vi "MainSimple.vi"() -> ()   [LabVIEW 2020]
uses:
  <vilib>/Platform/TimedLoop/XDataNode/timing_clust.ctl
  <vilib>/Platform/TimedLoop/XDataNode/nitl_modes.ctl
  <vilib>/Platform/TimedLoop/XDataNode/wakeup.ctl
  <vilib>/Platform/TimedLoop/XDataNode/loadnilvce.vi
  <vilib>/imath/engines/lvmath2/RunTimeEngine/Managers/WorkSpace/UID Generator.vi
  <vilib>/imath/engines/lvmath2/RunTimeEngine/RunTimeType/NIMS_RunTimeType_From StrictType (excl LVString).vi
  <instcachedir>/0/NIMS_RunTimeType_From StrictType (excl LVString)_283B1B2000484AAA8744D21CE97EA49F.lvgen/NIMS_RunTimeType_From StrictType (excl LVString)_283B1B2000484AAA8744D21CE97EA49F_000.vi
  <vilib>/imath/engines/lvmath2/RunTimeEngine/LocalVariableDefStatement/MC_LocalVariableDefStatement_Display.vi
  <vilib>/imath/engines/lvmath2/RunTimeEngine/BuiltInFunctions/round/NIMS_round(DBL-S).vi
  <vilib>/imath/engines/lvmath2/RunTimeEngine/RunTimeType/NIMS_RunTimeType_Set Source Original Bool.vi
  <vilib>/imath/engines/lvmath2/RunTimeEngine/Managers/SymbolTable/Clear UID.vi
  <vilib>/imath/engines/lvmath2/RunTimeEngine/NodeEndStatement/NIMS_NodeEndStatement_Output.vi
  <instcachedir>/0/NIMS_NodeEndStatement_Output_53EC0D466D134D7ABD903AC30B43404B.lvgen/NIMS_NodeEndStatement_Output_53EC0D466D134D7ABD903AC30B43404B_001.vi
  <instcachedir>/0/NIMS_NodeEndStatement_Output_53EC0D466D134D7ABD903AC30B43404B.lvgen/NIMS_NodeEndStatement_Output_53EC0D466D134D7ABD903AC30B43404B_010.vi
  <vilib>/imath/engines/lvmath2/RunTimeEngine/ErrorHandling/NIMS_Finalize Error.vi
  Global 2.vi
  <vilib>/platform/TimedLoop/XDataNode/XDataNode.xnode
  <vilib>/Platform/TimedLoop/XDataNode/XDNodeRunTimeDep.lvlib
  <vilib>/imath/engines/lvmath2/RunTimeEngine/Managers/SymbolTable/NIMS_WorkSpace.lvlib
panel:
  in  "AlphaX [rad]":dbl
  in  "AlphaY [rad]":dbl=1.57
  in  "SwimmerX [m]":dbl
  in  "SwimmerY [m]":dbl
  in  "SwimmerZ [m]":dbl
  in  "BMagnitude [T]":dbl=0.02
  out "LoopDuration [ms]":dbl=1.0
  out "Numeric":dbl=8325.0
  in  "Power On/Off":bool
  out "Power":bool
  out "VoltageSaturating":bool=TRUE
  out "Waveform Chart":dbl(graph)=-0.2668501091435667
  in  "ForwardRotationsPerSecond [Hz]":dbl=15.0
  in  "BackwardRotationsPerSecond [Hz]":dbl=-15.0
  in  "RotationsPerSecond [Hz]":dbl=-20.0
  in  "Bidirection":bool=TRUE
  out "RotationPerSecond[Hz]":dbl=94.24777499999999
  in  "Z_offset (m)":dbl
  in  "Search Rect (entire image)":T1={"Left"=256, "Top"=459, "Right"=496, "Bottom"=249, "Rotation"=0.0} {"Rotation" format="%.2f"; "Left" scale=0.0..1024.0; "Right" scale=0.0..1024.0}
  in  "Settings 4":T2={"Objects"=1, "Threshold"=95, "Reject Border"=FALSE, "Fill Holes"=FALSE, "Min Object Size"=TRUE, "Min Size"=25, "Max Object Size"=TRUE, "Max Size"=25000, "Show Search Area"=TRUE, "Show Center"=TRUE, "Show Bounding Box"=TRUE} {"Objects" items=["Bright Objects", "Dark Objects"]; "Threshold" min=1 max=999999999 step=1; "Max Size" min=1 max=999999999 step=1; "Min Size" min=1 max=999999999 step=1}
  out "Image 4":T3(plugin-control)
  in  "Settings 3":T2={"Objects"=1, "Threshold"=100, "Reject Border"=FALSE, "Fill Holes"=FALSE, "Min Object Size"=TRUE, "Min Size"=25, "Max Object Size"=TRUE, "Max Size"=25000, "Show Search Area"=FALSE, "Show Center"=TRUE, "Show Bounding Box"=TRUE} {"Objects" items=["Bright Objects", "Dark Objects"]; "Threshold" min=1 max=999999999 step=1; "Max Size" min=1 max=999999999 step=1; "Min Size" min=1 max=999999999 step=1}
  out "Image 3":T3(plugin-control)
  in  "Vision compensation":bool=TRUE
  out "Vision compensation active":bool=TRUE
  out "coordinates":cluster{dbl, dbl, dbl}(graph)={0.0146, -0.0144, 0.0736}
  out "camera rate":u32=29
  out "X":dbl=0.0146
  out "Y":dbl=-0.0144
  out "Z":dbl=0.0736
  out "Error_detection":bool
  out "Detection_Error":cdb
  out "Waveform Chart 2":dbl(graph)=27.12160697456251
  in  "TempSetpoint":dbl
  out "Temperature":dbl=27.12160697456251
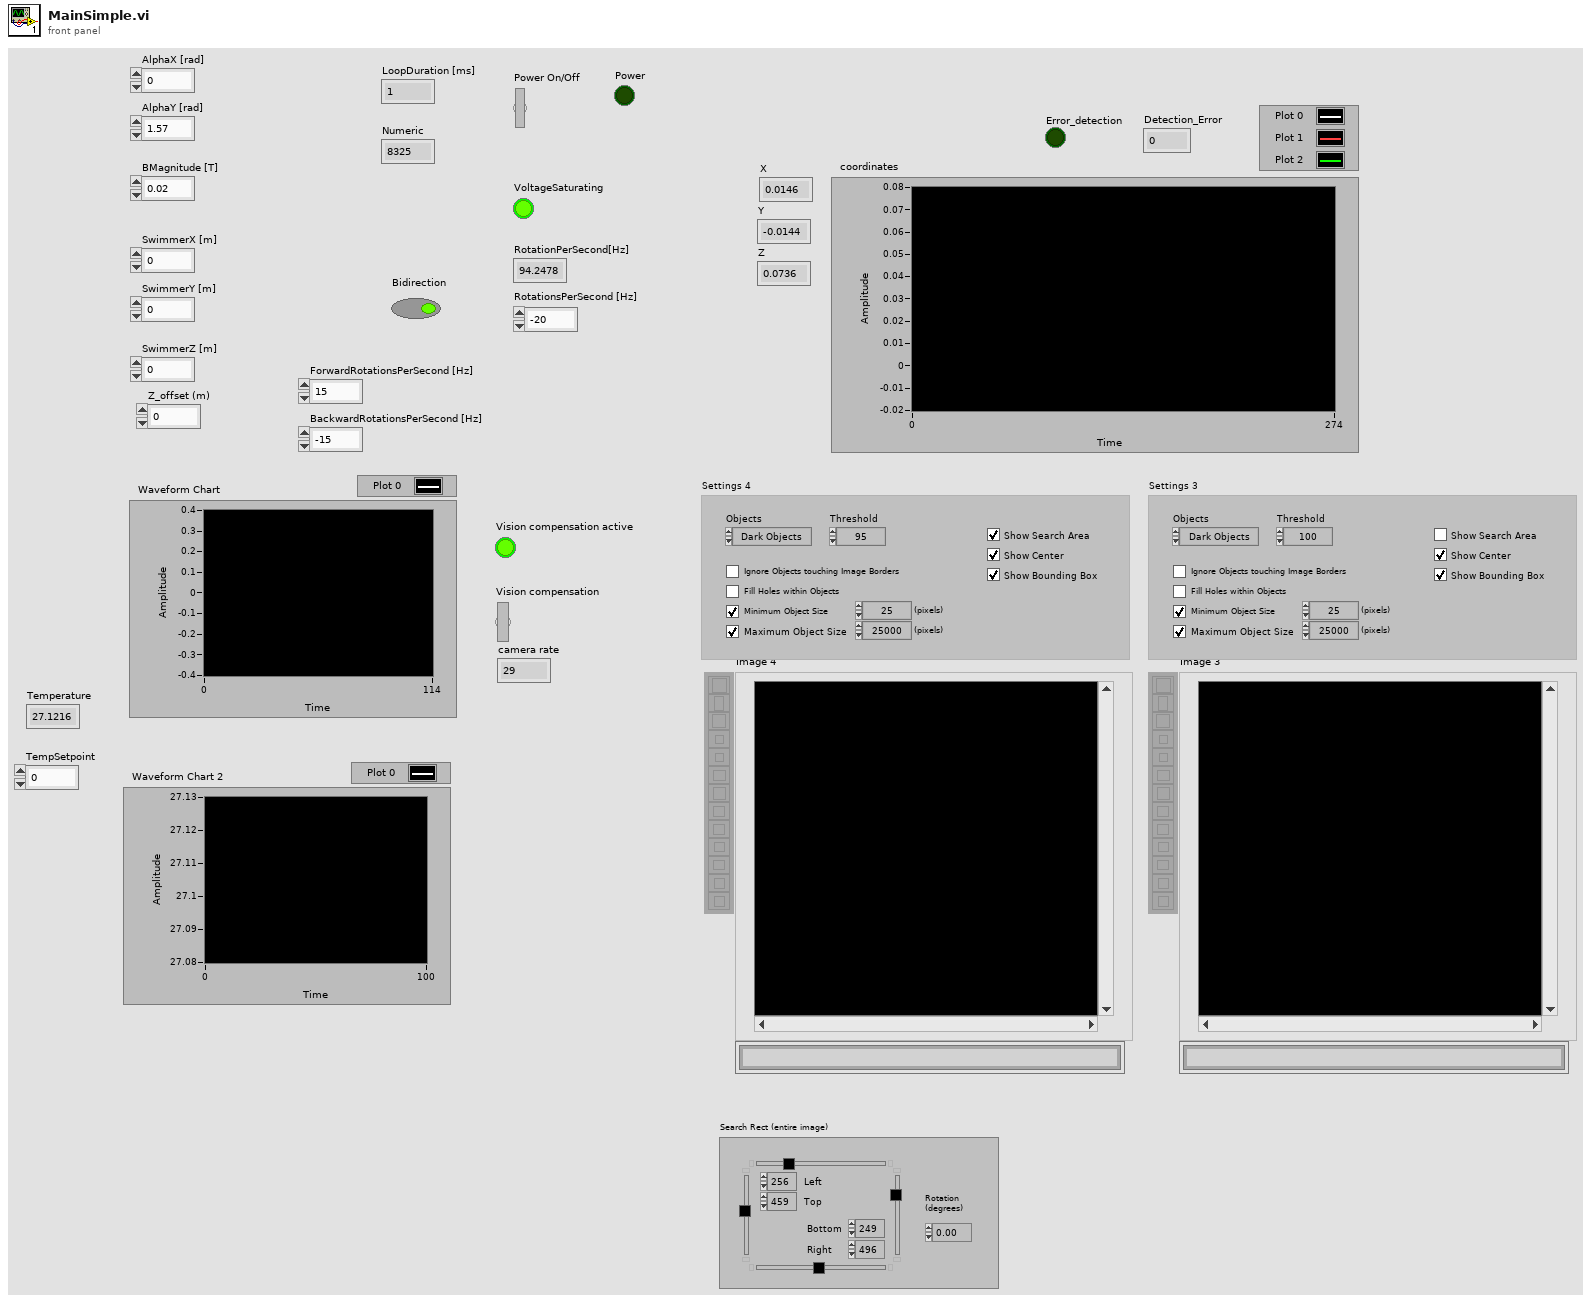
[diagram p1: front panel]
types:
  T1 = typedef "IMAQ Rectangle" = cluster{"Left":i32, "Top":i32, "Right":i32, "Bottom":i32, "Rotation":dbl}
  T2 = cluster{"Objects":u16, "Threshold":i32, "Reject Border":bool, "Fill Holes":bool, "Min Object Size":bool, "Min Size":i32, "Max Object Size":bool, "Max Size":i32, "Show Search Area":bool, "Show Center":bool, "Show Bounding Box":bool}
  T3 = typedef "IMAQ Image.ctl" = refnum<image>
  T4 = typedef "XDNodeRunTimeDep.lvlib/timing_clust.ctl" = cluster{"Expected End [f-1]":u64, "Actual End [f-1]":u64, "Finished Late? [f-1]":bool, "Expected End [i-1]":u64, "Actual End [i-1]":u64, "Finished Late? [i-1]":bool, "Expected Start [i]":u64, "Actual Start [i]":u64, "Expected Start [f]":u64, "Actual Start [f]":u64, "Source Name":string, "Structure Name":string, "Period":i64, "Deadline":i64, "Offset":i64, "Start":i64, "Priority":i32, "Timeout":i32, "Mode":T5, "Wakeup Reason":T6, "Error":errorcluster, "Source Type":string, "Secondary Source Type":string, "Global End Time":u64, "Global Start Time":u64, "Frame Duration":u64, "Iteration Duration":u64, "Assigned CPU":i32, "I/O Scan Engine Mode":u32}
  T5 = typedef "XDNodeRunTimeDep.lvlib/nitl_modes.ctl" = enum32{"No Change", "Process missed periods, maintain original phase", "Discard missed periods, maintain original phase", "Process missed periods, ignore original phase", "Discard missed periods, ignore original phase"}
  T6 = typedef "XDNodeRunTimeDep.lvlib/wakeup.ctl" = enum32{"Normal", "Aborted", "Asynchronous wakeup", "Timing source error", "Timed loop error", "Timeout"}
  T7 = cluster{"Object Center":cluster{"X":sgl, "Y":sgl}, "Bounding Box":cluster{"X Left":i32, "Y Top":i32, "X Right":i32, "Y Bottom":i32}, "Area":sgl, "Orientation":sgl, "Aspect Ratio":sgl, "Nb Holes":i32}[]
  T8 = cluster{"Objects[0]":cluster{"Object Center":cluster{"X":sgl, "Y":sgl}, "Bounding Box":cluster{"X Left":i32, "Y Top":i32, "X Right":i32, "Y Bottom":i32}, "Area":sgl, "Orientation":sgl, "Aspect Ratio":sgl, "Nb Holes":i32}, "Objects[1]":cluster{"Object Center":cluster{"X":sgl, "Y":sgl}, "Bounding Box":cluster{"X Left":i32, "Y Top":i32, "X Right":i32, "Y Bottom":i32}, "Area":sgl, "Orientation":sgl, "Aspect Ratio":sgl, "Nb Holes":i32}, "Objects[2]":cluster{"Object Center":cluster{"X":sgl, "Y":sgl}, "Bounding Box":cluster{"X Left":i32, "Y Top":i32, "X Right":i32, "Y Bottom":i32}, "Area":sgl, "Orientation":sgl, "Aspect Ratio":sgl, "Nb Holes":i32}, "Objects[3]":cluster{"Object Center":cluster{"X":sgl, "Y":sgl}, "Bounding Box":cluster{"X Left":i32, "Y Top":i32, "X Right":i32, "Y Bottom":i32}, "Area":sgl, "Orientation":sgl, "Aspect Ratio":sgl, "Nb Holes":i32}, "Objects[4]":cluster{"Object Center":cluster{"X":sgl, "Y":sgl}, "Bounding Box":cluster{"X Left":i32, "Y Top":i32, "X Right":i32, "Y Bottom":i32}, "Area":sgl, "Orientation":sgl, "Aspect Ratio":sgl, "Nb Holes":i32}, "Objects[5]":cluster{"Object Center":cluster{"X":sgl, "Y":sgl}, "Bounding Box":cluster{"X Left":i32, "Y Top":i32, "X Right":i32, "Y Bottom":i32}, "Area":sgl, "Orientation":sgl, "Aspect Ratio":sgl, "Nb Holes":i32}, "Objects[6]":cluster{"Object Center":cluster{"X":sgl, "Y":sgl}, "Bounding Box":cluster{"X Left":i32, "Y Top":i32, "X Right":i32, "Y Bottom":i32}, "Area":sgl, "Orientation":sgl, "Aspect Ratio":sgl, "Nb Holes":i32}, "Objects[7]":cluster{"Object Center":cluster{"X":sgl, "Y":sgl}, "Bounding Box":cluster{"X Left":i32, "Y Top":i32, "X Right":i32, "Y Bottom":i32}, "Area":sgl, "Orientation":sgl, "Aspect Ratio":sgl, "Nb Holes":i32}, "Objects[8]":cluster{"Object Center":cluster{"X":sgl, "Y":sgl}, "Bounding Box":cluster{"X Left":i32, "Y Top":i32, "X Right":i32, "Y Bottom":i32}, "Area":sgl, "Orientation":sgl, "Aspect Ratio":sgl, "Nb Holes":i32}}
  T9 = cluster{"Object Center":cluster{"X":sgl, "Y":sgl}, "Bounding Box":cluster{"X Left":i32, "Y Top":i32, "X Right":i32, "Y Bottom":i32}, "Area":sgl, "Orientation":sgl, "Aspect Ratio":sgl, "Nb Holes":i32}
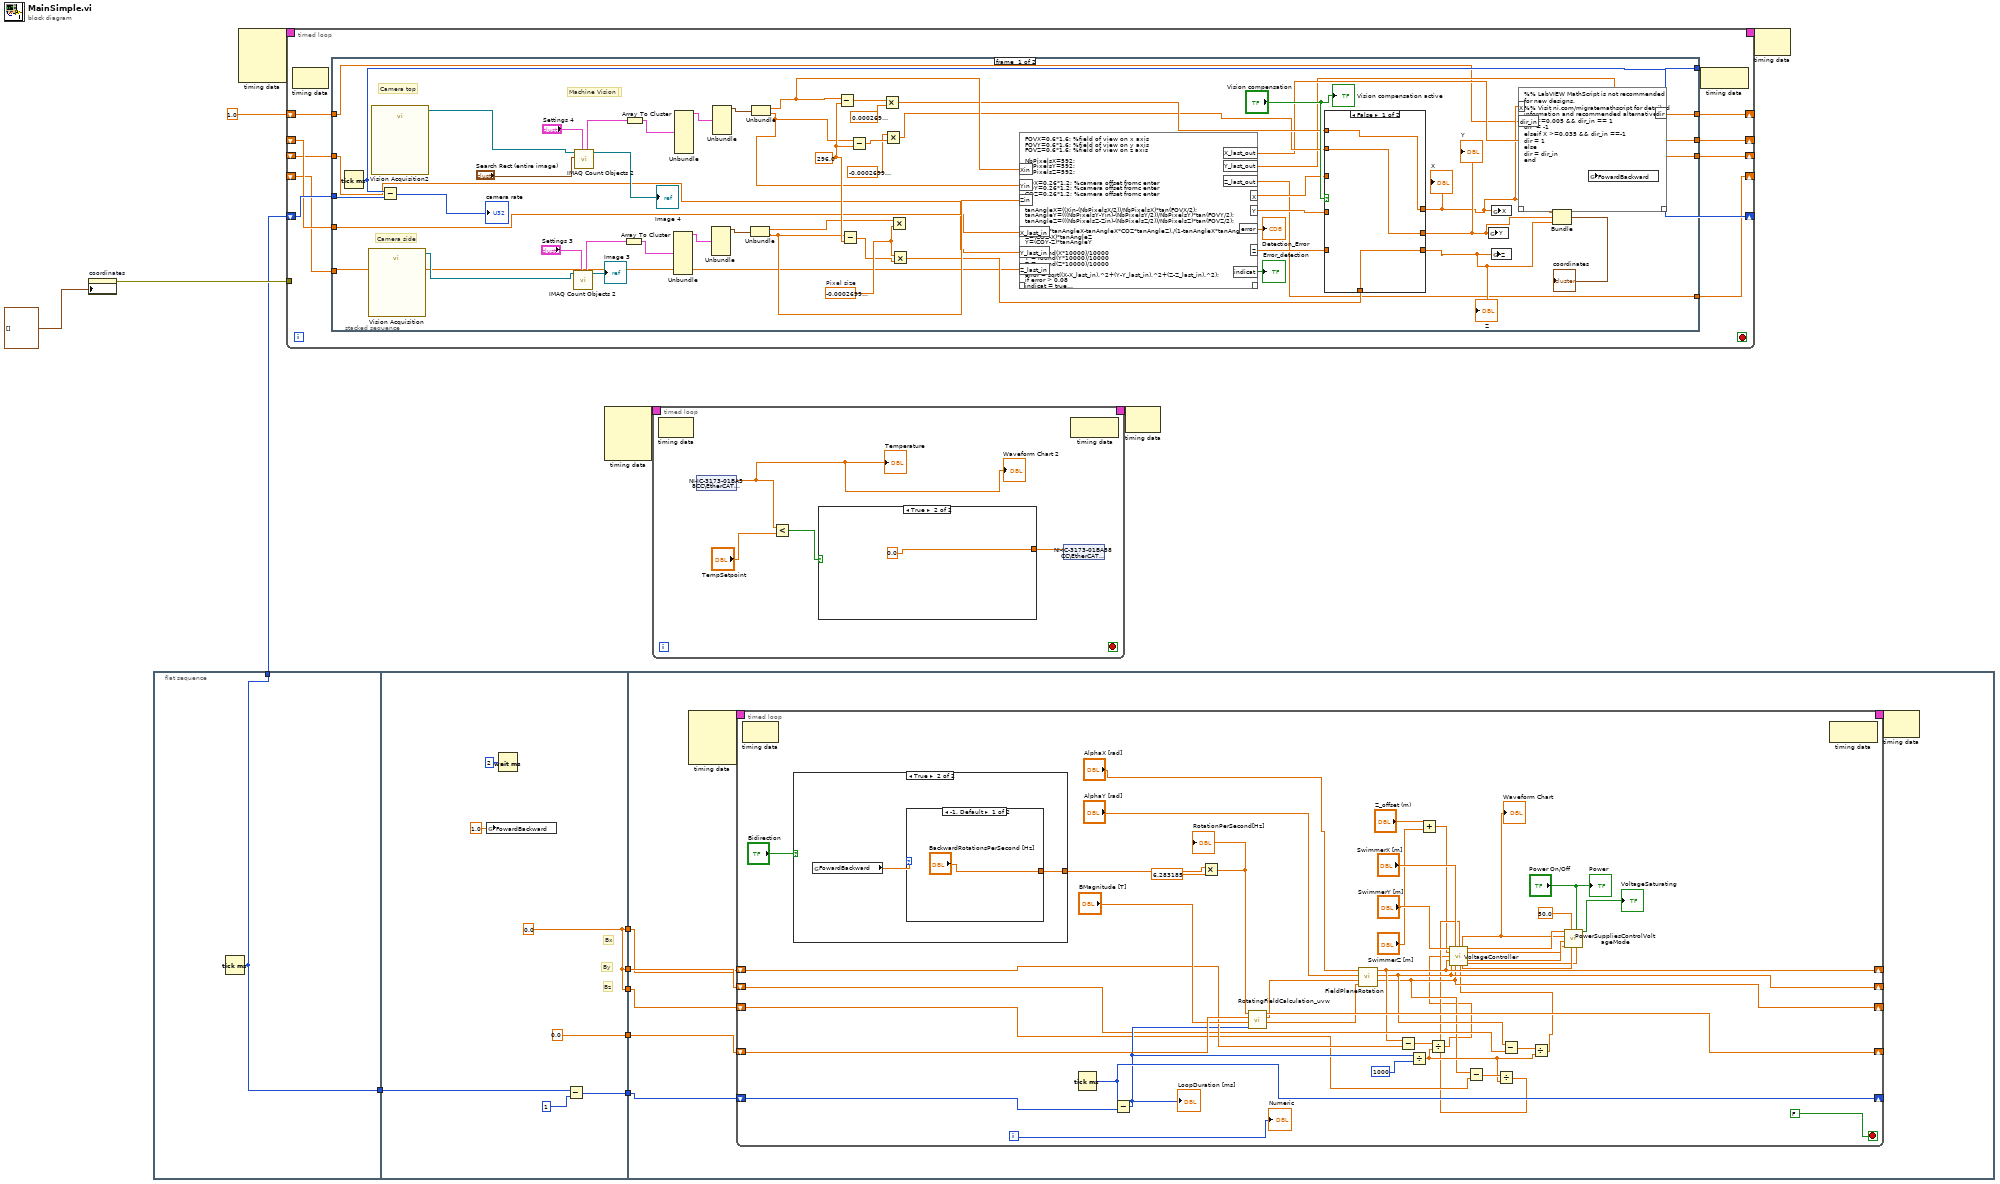
[diagram p0: block diagram]
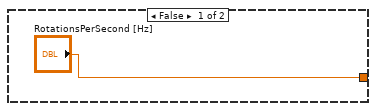
[diagram p2: hidden frame]
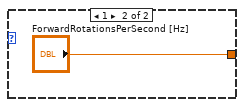
[diagram p3: hidden frame]
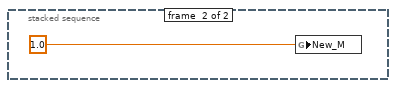
[diagram p5: hidden frame]
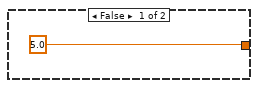
[diagram p6: hidden frame]
diagram:
  n1 = property on="coordinates" class="WFChart (strict)"("History Data"=cluster{dbl, dbl, dbl}[] []) -> (error out=w9:errorcluster)  [unwired: 2 in, 1 out]
  n2 = flat-sequence {
    tunnel: [w15] -> w3
    tunnel: [w15] -> w2
    tunnel: [0.0] -> w8
    tunnel: [w19] -> w7
    tunnel: [w20] -> w6
    tunnel: [w19] -> w5
    tunnel: [w19] -> w4
    tunnel: w3 -> [w17]
    tunnel: w8 -> [w26]
    tunnel: w7 -> [w23]
    tunnel: w6 -> [w27]
    tunnel: w5 -> [w24]
    tunnel: w4 -> [w25]
    frame #0 {
      n3 = Tick Count (ms)() -> (millisecond timer value=w15:u32)
    }
    frame #1 {
      w19 = 0.0
      # "Bz"
      # "By"
      # "Bx"
      n4 = global write "Global 2.vi" "FowardBackward"(1.0 ("FowardBackward")) -> ()
      n5 = Wait (ms)(milliseconds to wait=u32 2) -> ()  [unwired: 1 out]
      n6 = Subtract(x=w17, y=1) -> (x-y=w20:u32)
    }
    frame #2 {
      n7 = node-c288() -> (w29:T4)  [unwired: 4 in]
      n8 = timed-loop {
        shift-right: [w69] -> _
        shift-left: w26 -> [w72]
        timing: w29 -> [_]
        timing-out: [_] -> w28
        shift-right: [w67] -> _
        shift-left: w27 -> [w68]
        shift-right: [w43] -> _
        shift-left: w23 -> [w60]
        shift-right: [w42] -> _
        shift-left: w24 -> [w55]
        shift-right: [w41] -> _
        shift-left: w25 -> [w53]
        i -> [w66]
        stop <- FALSE stop-if-true
        n9 = node-c288() -> ()  [unwired: 1 in, 1 out]
        n10 = case shown="True" "Bidirection" {
          tunnel: ["RotationsPerSecond [Hz]" w75] -> w35
          frame False {
          }
          frame True {
            n11 = global read "Global 2.vi" "FowardBackward"() -> (w76:dbl)
            n12 = case shown="-1, Default" w76 {
              tunnel: ["BackwardRotationsPerSecond [Hz]" "ForwardRotationsPerSecond [Hz]"] -> w75
              frame -1, Default {
              }
              frame 1 {
              }
            }
          }
        }
        n13 = Tick Count (ms)() -> (millisecond timer value=w67:u32)
        n14 = Subtract(x=w67, y=w68) -> (x-y=w58:u32)
        "LoopDuration [ms]" <- w58
        n15 = Multiply(x=w35, y=6.283185) -> (x*y=w34:dbl)
        "RotationPerSecond[Hz]" <- w34
        n16 = call "RotatingFieldCalculation_uvw.vi"("Time Step (ms)"=w58, "Flux density magnitude (T)"="BMagnitude [T]", "Previous Field Angle (rad)"=w72, "Omega (rad/s)"=w34) -> ("Bv (T)"=w63:sgl, "Bu (T)"=w44:sgl, "New Field Angle (rad)"=w69:sgl)  [unwired: 5 in]
        n17 = call "FieldPlaneRotation.vi"("Bv (T)"=w63, "Bu (T)"=w44, "AlfaY (rad)"="AlphaY [rad]", "AlfaX (rad)"="AlphaX [rad]") -> ("Bz (T)"=w41:dbl, "By (T)"=w42:dbl, "Bx (T)"=w43:dbl)  [unwired: 5 in]
        n18 = Subtract(x=w43, y=w60) -> (x-y=w59:dbl)
        n19 = Divide(x=w58, y=1000) -> (x/y=w52:dbl)
        n20 = Add(x="Z_offset (m)", y="SwimmerZ [m]") -> (x+y=w31:dbl)
        n21 = Divide(x=w59, y=w52) -> (x/y=w37:dbl)
        n22 = Subtract(x=w41, y=w53) -> (x-y=w54:dbl)
        n23 = Divide(x=w54, y=w52) -> (x/y=w38:dbl)
        n24 = Subtract(x=w42, y=w55) -> (x-y=w56:dbl)
        n25 = Divide(x=w56, y=w52) -> (x/y=w39:dbl)
        n26 = call "VoltageController.vi"("Y (m)"="SwimmerY [m]", "X (m)"="SwimmerX [m]", "dBzdt"=w38, "Z (m)"=w31, "dBxdt"=w37, "Bx [T]"=w43, "By [T]"=w42, "Bz [T]"=w41, "dBydt"=w39) -> ("XN"=w36:dbl, "XP"=w40:dbl, "YN"=w50:dbl, "YP"=w51:dbl, "ZP"=w49:dbl, "ZN"=w48:dbl)  [unwired: 1 in]
        "Waveform Chart" <- w36
        n27 = call "PowerSuppliesControlVoltageMode.vi"("Z-"=w48, "OnOff"="Power On/Off", "Z+"=w49, "Max Voltage (V)"=50.0, "Y-"=w50, "Y+"=w51, "X-"=w36, "X+"=w40) -> ("Saturating"=→"VoltageSaturating":bool)  [unwired: 3 in]
        n28 = node-c288() -> ()  [unwired: 1 in, 1 out]
        "Numeric" <- w66
        "Power" <- "Power On/Off"
      }
      n29 = node-c288(w28) -> ()  [unwired: 1 out]
    }
  }
  n30 = node-c288() -> (w12:T4)  [unwired: 4 in]
  n31 = timed-loop {
    timing: w12 -> [_]
    timing-out: [_] -> w11
    tunnel: w9 -> [_]
    shift-right: [w91] -> _
    shift-left: w2 -> [w92]
    shift-right: [w90] -> _
    shift-left: _ -> [w87]
    shift-right: [w89] -> _
    shift-left: _ -> [w86]
    shift-right: [w88] -> _
    shift-left: _ -> [w85]
    shift-right: [w84] -> _
    shift-left: 1.0 ("dir") -> [w83]
    stop <- _ stop-if-true
    n32 = node-c288() -> ()  [unwired: 1 in, 1 out]
    n33 = stacked-sequence {
      tunnel: w92 -> [w107 _]
      tunnel: [w106 _] -> w91
      tunnel: [w102 _] -> w90
      tunnel: [w101 _] -> w89
      tunnel: [w100 _] -> w88
      tunnel: w87 -> [w99 _]
      tunnel: w86 -> [w98 _]
      tunnel: w85 -> [w97 _]
      tunnel: [w94 _] -> w84
      tunnel: w83 -> [w93 _]
      frame #0 {
        w123 = 296.0
        w127 = sgl -0.00027  # Pixel size
        # "Machine Vision"
        # "Camera top"
        # "Machine Vision"
        # "Camera side"
        n34 = Tick Count (ms)() -> (millisecond timer value=w106:u32)
        n35 = call "Vision Acquisition"() -> ("Image Out"=w129:T3)  [unwired: 25 in, 2 out]
        n36 = call "Vision Acquisition2"() -> ("Image Out"=w140:T3)  [unwired: 25 in, 2 out]
        n37 = Subtract(x=w106, y=w107) -> (x-y=→"camera rate":u32)
        n38 = call "IMAQ Count Objects 2"("Settings"="Settings 3", "Image"=w129) -> ("Image Out"=→"Image 3":T3, "Objects"=w133:T7)  [unwired: 5 in, 3 out]
        n39 = call "IMAQ Count Objects 2"("Settings"="Settings 4", "Search Rect (entire image)"="Search Rect (entire image)", "Image"=w140) -> ("Image Out"=→"Image 4":T3, "Objects"=w139:T7)  [unwired: 4 in, 3 out]
        n40 = Array To Cluster(array=w133) -> (cluster=w132:T8)
        n41 = Array To Cluster(array=w139) -> (cluster=w138:T8)
        n42 = Unbundle(w132) -> ("Objects[0]"=w131:T9)  [unwired: 8 out]
        n43 = Unbundle(w138) -> ("Objects[0]"=w137:T9)  [unwired: 8 out]
        n44 = Unbundle(w131) -> ("Object Center"=w130:cluster{"X":sgl, "Y":sgl})  [unwired: 5 out]
        n45 = Unbundle(w137) -> ("Object Center"=w136:cluster{"X":sgl, "Y":sgl})  [unwired: 5 out]
        n46 = Unbundle(w130) -> ("X"=w121:sgl, "Y"=w118:sgl)
        n47 = Unbundle(w136) -> ("X"=w120:sgl, "Y"=w119:sgl)
        n48 = Subtract(x=w120, y=w123) -> (x-y=w126:dbl)
        n49 = Subtract(x=w118, y=w123) -> (x-y=w124:dbl)
        n50 = Subtract(x=w119, y=w123) -> (x-y=w125:dbl)
        n51 = Multiply(x=w126, y=sgl 0.00027) -> (x*y=w114:dbl)
        n52 = Multiply(x=sgl -0.00027 ("y"), y=w125) -> (x*y=w113:dbl)
        n53 = Multiply(x=w121, y=w127) -> ()  [unwired: 1 out]
        n54 = Multiply(x=w127, y=w124) -> (x*y=w112:dbl)
        n55 = mathscript code="FOVX=0.6*1.6; %field of view on x axis\nFOVY=0.6*1.6; %field of view on y axis\nFOVZ=0.6*1.6; %field of view on z axis\n\nNbPixelsX=592;\nNbPixelsY=592;\nNbPixelsZ=592;\n\nCOX=0.26*1.2; %camera offset fromc enter\nCOY=0.26*1.2; %camera offset fromc enter\nCOZ=0.26*1.2; %camera offset fromc enter\n\n\ntanAngleX=((Xin-(NbPixelsX/2))/NbPixelsX)*tan(FOVX/2);\ntanAngleY=(((NbPixelsY-Yin)-(NbPixelsY/2))/NbPixelsY)*tan(FOVY/2);\ntanAngleZ=(((NbPixelsZ-Zin)-(NbPixelsZ/2))/NbPixelsZ)*tan(FOVZ/2);\n\nX=(COX*tanAngleX-tanAngleX*COZ*tanAngleZ)./(1-tanAngleX*tanAngleY)\nZ=(COZ-X)*tanAngleZ\nY=(COY-Z)*tanAngleY\n\nX = round(X*10000)/10000\nY = round(Y*10000)/10000\nZ = round(Z*10000)/10000\n\nerror = sqrt((X-X_last_in).^2+(Y-Y_last_in).^2+(Z-Z_last_in).^2);\nif error > 0.08\nindicat = true\nX = X_last_in\nY=Y_last_in\nZ= Z_last_in\nelse\nindicat = false\nend\n\nX_last_out = X\nY_last_out = Y\nZ_last_out = Z"("Xin"=w120, "Yin"=w119, "Zin"=w118, "X_last_in"=w99, "Y_last_in"=w98, "Z_last_in"=w97) -> ("X"=w105:dbl, "Y"=w116:dbl, "Z"=w115:dbl, "indicat"=→"Error_detection":bool, "error"=→"Detection_Error":dbl, "X_last_out"=w102:dbl, "Y_last_out"=w101:dbl, "Z_last_out"=w100:dbl)  [unwired: 1 in, 1 out]
        n56 = case shown="False" "Vision compensation" {
          tunnel: [w256 w259] -> w95
          tunnel: w105 -> [_ w259]
          tunnel: [w255 w258] -> w110
          tunnel: w116 -> [_ w258]
          tunnel: [w254 w257] -> w109
          tunnel: w115 -> [_ w257]
          tunnel: w114 -> [w256 _]
          tunnel: w113 -> [w255 _]
          tunnel: w112 -> [w254 _]
          frame False {
          }
          frame True {
          }
        }
        "X" <- w95
        "Y" <- w110
        "Z" <- w109
        n57 = global write "Global 2.vi" "Y"(w110) -> ()
        n58 = global write "Global 2.vi" "Z"(w109) -> ()
        n59 = global write "Global 2.vi" "X"(w95) -> ()
        n60 = mathscript code="%% LabVIEW MathScript is not recommended for new designs.\n%% Visit ni.com/migratemathscript for detailed information and recommended alternatives.\nif X <=0.005 && dir_in == 1\ndir  = -1\nelseif X >=0.035 && dir_in ==-1\ndir = 1\nelse\ndir = dir_in\nend"("X"=w95, "dir_in"=w93) -> ("dir"=w94:dbl)  [unwired: 1 in, 1 out]
        n61 = Bundle("X"=w95, "Y"=w110, "Z"=w109) -> (→"coordinates":cluster{"X":dbl, "Y":dbl, "Z":dbl})  [unwired: 1 in]
        n62 = global write "Global 2.vi" "FowardBackward"(w94) -> ()
        "Vision compensation active" <- "Vision compensation"
      }
      frame #1 {
        n63 = global write "Global 2.vi" "New_M"(1.0 ("New_M")) -> ()
      }
    }
    n64 = node-c288() -> ()  [unwired: 1 in, 1 out]
  }
  n65 = node-c288() -> (w14:T4)  [unwired: 4 in]
  n66 = timed-loop {
    timing: w14 -> [_]
    timing-out: [_] -> w13
    stop <- _ stop-if-true
    n67 = node-c288() -> ()  [unwired: 1 in, 1 out]
    n68 = shared-variable "NI-IC-3173-01BA58CC\\EtherCAT Master\\Device\\Mod3\\TC7"() -> (w682:dbl)  [unwired: 1 in, 1 out]
    "Temperature" <- w682
    "Waveform Chart 2" <- w682
    n69 = Less?(x=w682, y="TempSetpoint") -> (x < y?=w683:bool)
    n70 = case shown="True" w683 {
      tunnel: [5.0 0.0] -> w685
      frame False {
      }
      frame True {
      }
    }
    n71 = shared-variable "NI-IC-3173-01BA58CC\\EtherCAT Master\\Device\\Mod2\\AO3"(w685) -> ()  [unwired: 1 in, 1 out]
    n72 = node-c288() -> ()  [unwired: 1 in, 1 out]
  }
  n73 = node-c288(w13) -> ()  [unwired: 1 out]
  n74 = node-c288(w11) -> ()  [unwired: 1 out]
